vi "FEA_Model_eigh.vi"(2 "Stiffness":T2=array398x398[158404 elements], 3 "Mass":T2=array398x398[158404 elements]) -> (0 "Eigenvectors":T1, 1 "Eigenvalues":dbl[](array[numeric])=[57324.18969647021, 2340326.773945595, 18842923.72259714, 73907396.15765077, 205349469.9890637, 464384954.46519357, 915784527.7517059, 1637891666.3815625, 2722632472.8846316, 4275515279.325833, 6415624969.193008, 9275613725.040789, 13001692027.533115, 17753614901.423603, 23704669002.43506, 31041656469.031185, 39964879816.702194, 50688121841.734344, 63438626980.45474, 78457079813.79535, 95997581988.6117, 116327626980.8429, 139728073712.95016, 166493117567.83093, 196930257577.8631, 231360266083.93283, 270117150347.5564, 313548113007.63965, 362013512558.3495, 415886816618.86835, 475554556190.9326, 541416269080.44867, 613884450915.5371, 693384492440.8652, 780354619231.5298, 875245824616.3925, 978521802056.0394, 1090658872603.2037, 1212145906834.1458, 1343484252719.8376, 1485187656790.9333, 1637782190349.3826, 1801806169115.9978, 1977810088703.2822, 2166356563521.263, 2368020279576.7393, 2583387949314.072, 2813058314874.0273, 3057642138480.3125, 3317762272596.151, 3594053718336.367, 3887163785997.987, 4197752261882.221, 4526491651970.804, 4874067513276.024, 5241178814916.885, 5628538423739.423, 6036873586904.214, 6466926533285.593, 6919455109633.198, 7395233418375.991, 7895052518633.381, 8419721022281.91, 8970065740329.162, 9546932183309.566, 10151184976956.836, 10783708168112.809, 11445405362881.02, 12137199736136.256, 12860033905237.787, 13614869658614.9, 14402687594584.03, 15224486657077.748, 16081283685922.305, 16974112875378.494, 17904025312459.027, 18872088515772.46, 19879386048501.082, 20927017174127.316, 22016096680017.48, 23147754605824.973, 24323136280774.438, 25543402207235.453, 26809728151436.02, 28123305260617.945, 29485340132701.55, 30897055118985.55, 32359688389607.785, 33874494307453.61, 35442743543535.75, 37065723428079.62, 38744738172156.125, 40481109134113.02, 42276175110607.94, 44131292583528.08, 46047835996272.5, 48027198000868.24, 50070789813727.125, 52180041323067.2, 54356401488425.04, 56601338536617.86, 58916340277289.164, 61302914288499.9, 63762588237758.92, 66296910106615.64, 68907448494118.57, 71595792781124.61, 74363553605060.06, 77212362869927.75, 80143874223014.53, 83159763143655.97, 86261727362292.8, 89451487044580.45, 92730785139576.97, 96101387581216.72, 99565083564223.05, 103123685940825.9, 106779031382507.62, 110532980612702.23, 114387418849248.23, 118344256036173.22, 122405426997758.4, 126572891821172.61, 130848636244115.92, 135234671689682.58, 139733035655498.38, 144345792100433.72, 149075031433285.25, 153922871075542.84, 158891455479439.34, 163982956480768.84, 169199573475812.34, 174543533707346.38, 180017092335585.28, 185622532792031.34, 191362166857426.9, 197238334788276.12, 203253405444754.75, 209409776517619.72, 215709874304784.66, 222156154069208.78, 228751099707482.3, 235497223932908.28, 242397067968510.94, 249453201536901.44, 256668222541015.97, 264044756509003.9, 271585456633238.9, 279293002803623.84, 287170101163036.5, 295219483465438.3, 303443905837277.0, 311846147750000.3, 320429011027087.4, 329195317731802.3, 338147908909055.6, 347289641907544.4, 356623388410250.94, 366152031059008.56, 375878460267907.06, 385805570055176.7, 395936253310089.2, 406273396574390.25, 416819872989033.06, 427578534875682.75, 438552204727703.7, 449743664146515.0, 461155641179870.3, 472790794899573.8, 484651696941848.0, 496740809491096.75, 509060457743455.1, 521612798188417.4, 534399778013495.8, 547423085293601.1, 560684088738315.8, 574183760327140.4, 587922580396813.2, 601900415114552.5, 616116360605280.6, 630568543874100.6, 645253859540316.9, 660167626918822.2, 675303132784373.4, 690651013328068.8, 706198414871018.5, 721927829689407.6, 737815465900471.9, 753828924314225.6, 769923840620793.5, 786038959565398.6, 802088806916336.8, 817952685669791.2, 833458094327715.1, 848355989909978.5, 862285094163182.1, 874723979810274.4, 884934454759382.6, 891910721202564.9, 909937758009993.9, 1088649957669511.5, 1095929339913804.2, 1107243458087227.0, 1121756328301595.8, 1138735358718552.5, 1157621907777862.0, 1178017168747350.5, 1199643793566512.8, 1222309967457149.8, 1245882489699087.8, 1270268168089524.2, 1295401343138600.0, 1321235544252224.0, 1347737903117768.5, 1374885348788757.8, 1402661989863789.2, 1431057286622201.2, 1460064746546831.5, 1489680993950089.8, 1519905082534945.5, 1550737994761724.8, 1582182257998151.8, 1614241668685292.0, 1646921060537150.2, 1680226148424105.5, 1714163389761557.8, 1748739881364360.0, 1783963284443140.0, 1819841754513909.2, 1856383893949433.0, 1893598703140482.5, 1931495560617783.8, 1970084181188089.0, 2009374606593172.2, 2049377179154158.2, 2090102534312290.5, 2131561584710583.0, 2173765511769162.8, 2216725756001909.2, 2260454022921744.0, 2304962257802260.0, 2350262662104751.5, 2396367679858359.0, 2443289994506425.0, 2491042538145654.5, 2539638477752609.5, 2589091223110994.0, 2639414425741431.5, 2690621980195449.0, 2742728014198788.5, 2795746909521275.5, 2849693283122604.5, 2904582000884634.5, 2960428176599958.0, 3017247172346058.0, 3075054600401521.0, 3133866320115410.0, 3193698455472225.5, 3254567377770020.0, 3316489717268121.5, 3379482366333986.5, 3443562484473190.5, 3508747489513928.0, 3575055058991141.5, 3642503150532603.5, 3711109985247617.0, 3780894050780673.0, 3851874110868095.5, 3924069197675197.0, 3997498619309947.0, 4072181948136458.5, 4148139032673850.5, 4225389990004321.5, 4303955202212639.0, 4383855312095715.5, 4465111224072673.0, 4547744102297698.0, 4631775350664416.0, 4717226623097733.0, 4804119794497124.0, 4892476974485616.0, 4982320474716886.0, 5073672824628966.0, 5166556710025747.0, 5260995018741689.0, 5357010757898036.0, 5454627101037715.0, 5553867318557252.0, 5654754763902227.0, 5757312872953094.0, 5861565112298633.0, 5967534973674746.0, 6075245924618110.0, 6184721388627444.0, 6295984688289724.0, 6409059065152816.0, 6523967566492697.0, 6640733083830347.0, 6759378238496308.0, 6879925407135902.0, 7002396594936877.0, 7126813462759133.0, 7253197219567342.0, 7381568621883960.0, 7511947848772199.0, 7644354500461822.0, 7778807495332094.0, 7915325036692032.0, 8053924481767733.0, 8194622371288402.0, 8337434242455708.0, 8482374622991416.0, 8629456861392506.0, 8778693177437564.0, 8930094418013950.0, 9083670049729966.0, 9239428002705814.0, 9397374623096130.0, 9557514519724968.0, 9719850434335504.0, 9884383166941636.0, 1.0051111375992904e+16, 1.0220031564066164e+16, 1.0391137844680336e+16, 1.0564421769754534e+16, 1.0739872348790558e+16, 1.0917475693677812e+16, 1.109721502126191e+16, 1.127907039239082e+16, 1.1463018676336632e+16, 1.1649033184678588e+16, 1.1837083736591752e+16, 1.2027136247875668e+16, 1.2219152761289788e+16, 1.2413091157942396e+16, 1.260890496424712e+16, 1.2806543231097902e+16, 1.300595034102125e+16, 1.3207065816981184e+16, 1.3409824100383668e+16, 1.3614154409670614e+16, 1.3819980579927174e+16, 1.4027220917039866e+16, 1.4235787888765144e+16, 1.444558816577803e+16, 1.465652230809223e+16, 1.4868484707567944e+16, 1.5081363358574598e+16, 1.5295039933221446e+16, 1.550938942058045e+16, 1.5724280227036932e+16, 1.5939574000401302e+16, 1.6155125634801468e+16, 1.6370783114606408e+16, 1.6586387752006862e+16, 1.680177378317798e+16, 1.7016768880520596e+16, 1.7231193829226492e+16, 1.7444862864139334e+16, 1.7657583633898862e+16, 1.786915748292412e+16, 1.807937953400631e+16, 1.828803903285659e+16, 1.849491946531884e+16, 1.869979902209041e+16, 1.8902450850069396e+16, 1.910264334910452e+16, 1.9300140832028e+16, 1.9494703748234612e+16, 1.96860893461687e+16, 1.9874052173444412e+16, 2.0058344603829756e+16, 2.0238717520685452e+16, 2.0414921126128804e+16, 2.0586705176648892e+16, 2.0753820215894624e+16, 2.091601815021323e+16, 2.10730528717859e+16, 2.122468133385367e+16, 2.1370664150481036e+16, 2.1510766589189344e+16, 2.164475925432977e+16, 2.1772419242137296e+16, 2.189353050374903e+16, 2.2007885236471344e+16, 2.2115284355411816e+16, 2.221553847521475e+16, 2.230846857910318e+16, 2.2393906855337016e+16, 2.2471697376480412e+16, 2.254169702884662e+16, 2.2603775716234956e+16, 2.2657817239183124e+16, 2.270371987785269e+16, 2.2741396645419244e+16, 2.2770775777903908e+16, 2.2791801241660108e+16, 2.2804432673463e+16] min=0.0 max=127.0 format="%.2f")   [LabVIEW 2021, in "FEA_Model.lvclass"]
uses:
  FEA_Model.lvclass
  <vilib>/Analysis/Matrix/Datatypes/RealMatrix.ctl
  <vilib>/Analysis/Matrix/Datatypes/ComplexMatrix.ctl
  <vilib>/Analysis/7linalg.llb/Real Generalized Eigenvalues and Vectors.vi
  <vilib>/Analysis/7linalg.llb/Real Transpose Matrix.vi
  <vilib>/Analysis/baseanly.llb/Real A x B.vi
  <vilib>/Analysis/Matrix/Numeric/Complex/Complex To Cartesian - CM.vi
  <vilib>/Analysis/Matrix/Numeric/Absolute Value/Absolute Value - RM.vi
  <vilib>/Analysis/NI_AALPro.lvlib
  <vilib>/Analysis/NI_AALBase.lvlib
  <vilib>/Analysis/Matrix/NI_Matrix.lvlib
panel:
  # "Documentation\n\nLorem Ipsum"
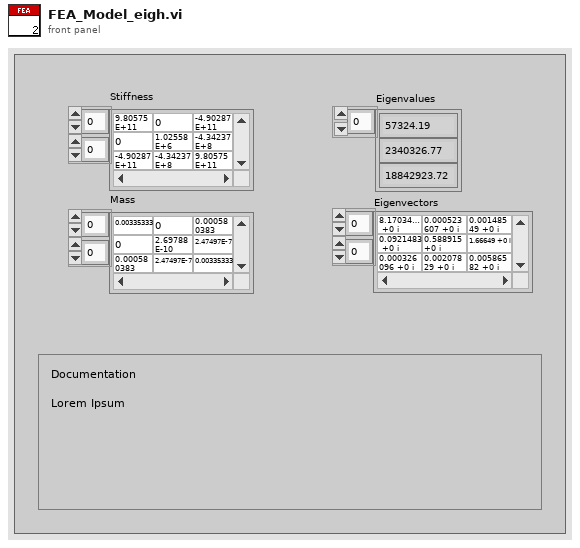
[diagram p1: front panel]
types:
  T1 = typedef "NI_Matrix.lvlib/ComplexMatrix.ctl" = cdb[][]
  T2 = typedef "NI_Matrix.lvlib/RealMatrix.ctl" = dbl[][]
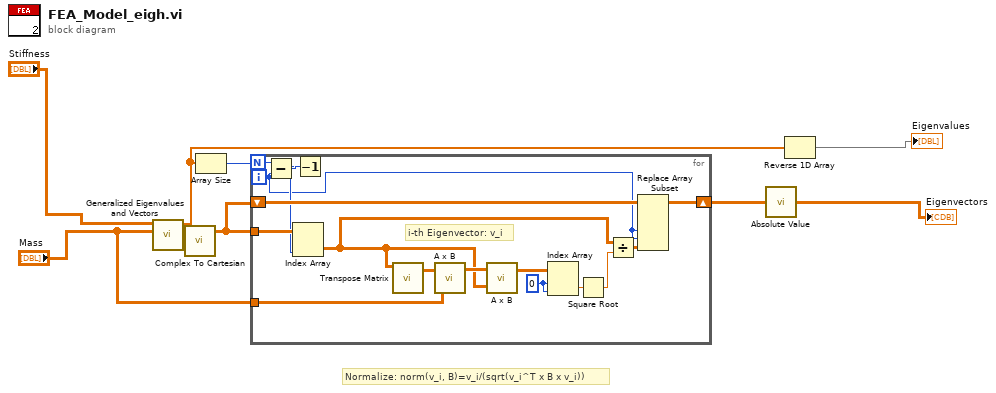
[diagram p0: block diagram]
diagram:
  # "Normalize: norm(v_i, B)=v_i/(sqrt(v_i^T x B x v_i))"
  n1 = call-poly <vilib>:"Generalized Eigenvalues and Vectors.vi"("B"="Mass", "A"="Stiffness") -> ("Eigenvectors"=w6:T1, "Eigenvalues"=w7:cdb[])  [unwired: 4 in, 1 out]
  n2 = call-poly <vilib>:"Complex To Cartesian.vi"("Complex Matrix R + Ii"=w6) -> ("Real Matrix R"=w5:T2)  [unwired: 1 out]
  n3 = Array Size(array=w7) -> (size(s)=w9:i32)
  n4 = for {
    N: w9 -> [w14]
    tunnel: w5 -> [w25]
    tunnel: "Mass" -> [w18]
    shift-right: [w22] -> w8
    shift-left: w5 -> [w23]
    i -> [w10]
    w15 = 0 ("index (row)")
    # "i-th Eigenvector: v_i"
    n5 = Subtract(x=w14, y=w10) -> (x-y=w12:i32)
    n6 = Decrement(x=w12) -> (x-1=w11:i32)
    n7 = Index Array(array=w25, index (col)=w11) -> (element=w13:T2)  [unwired: 1 in]
    n8 = call-poly <vilib>:"Transpose Matrix.vi"("Input Matrix"=w13) -> ("Matrix Transpose"=w21:T2)  [unwired: 9 in, 1 out]
    n9 = call-poly <vilib>:"A x B.vi"("B"=w18, "A"=w21) -> ("A x B"=w19:T2)  [unwired: 1 out]
    n10 = call-poly <vilib>:"A x B.vi"("B"=w13, "A"=w19) -> ("A x B"=w17:T2)  [unwired: 1 out]
    n11 = Index Array(array=w17, index (row)=w15, index (col)=w15) -> (element=w16:dbl)
    n12 = Square Root ("Square Root.vi")(x=w16) -> (sqrt(x)=w24:dbl)
    n13 = Divide(x=w13, y=w24) -> (x/y=w20:T2)
    n14 = Replace Array Subset(array=w23, new element=w20, index (dim 2)=w10, index (dim 3)=w10) -> (w22:T2)  [unwired: 2 in]
  }
  n15 = call-poly <vilib>:"Absolute Value.vi"("Real Matrix A"=w8) -> ("|A|"=→"Eigenvectors":T2)
  n16 = Reverse 1D Array(array=w7) -> (reversed array=→"Eigenvalues":cdb[])
